vi "Read_Variable2.vi"(0 "DDE Service name":string="ROBCOMM", 1 "Variable name":string) -> (2 "Variable name":string, 3 "Value":dbl, 4 "Error?":bool)   [LabVIEW 2012]
panel:
  in  "Command":string="VARIABLE"
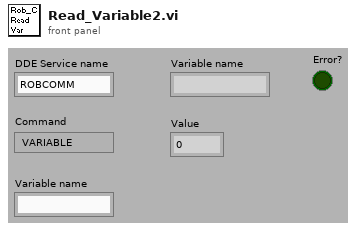
[diagram p1: front panel]
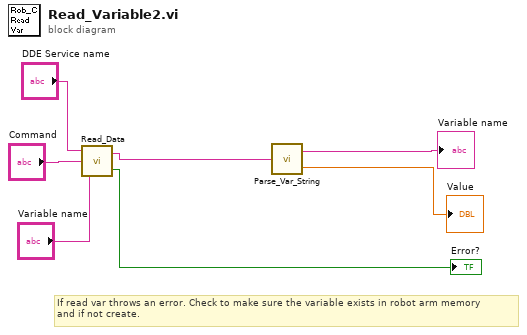
[diagram p0: block diagram]
diagram:
  # "If read var throws an error. Check to make sure the variable exists in robot arm memory \nand if not create."
  n1 = call <userlib>:"Read_Data.vi"("item"="Variable name", "topic"="Command", "service"="DDE Service name") -> ("Error?"=→"Error?":bool, "data"=w5:string)
  n2 = call <userlib>:"Parse_Var_String.vi"("Input"=w5) -> ("Variable name"=→"Variable name":string, "Value"=→"Value":dbl)
